vi "shared-dependency-declareself-test.vi"(8 "error in (no error)":errorcluster) -> (0 "error out":errorcluster)   [LabVIEW 2013]
uses:
  _test-support-SMOs/SMO.SelfTerminatingOverride/SMO.SelfTerminatingOverride.lvclass
  src/SMO/SMO.lvclass
  <vilib>/addons/_JKI Toolkits/Caraya/classes/Assert/Assert.lvclass
  <vilib>/addons/_JKI Toolkits/Caraya/classes/Test/Test.lvclass
  src/Registry/Registry-SMO.lvclass
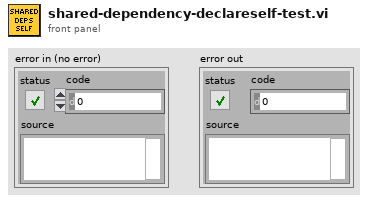
[diagram p1: front panel]
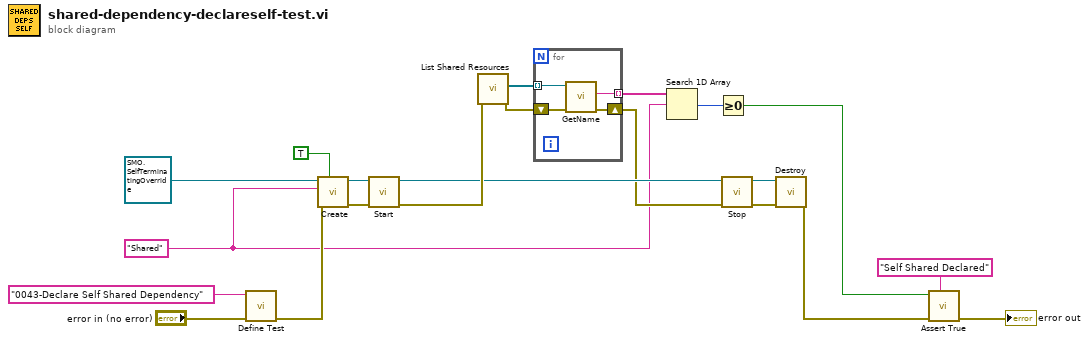
[diagram p0: block diagram]
diagram:
  w4 = "Shared" ("Subsystem Name (optional)")
  n1 = call <vilib>:"Define Test.vi"("error in (no error)"="error in (no error)", "Label (VI Title)"="0043-Declare Self Shared Dependency") -> ("error out"=w13:errorcluster)  [unwired: 9 in]
  n2 = call "Create.vi"("Shared Resource (F)"=TRUE, "error in (no error)"=w13, "Subsystem Name (optional)"=w4, "SMO"=refnum<class "SMO.SelfTerminatingOverride.lvclass"> refnum ("SMO.SelfTerminatingOverride.lvclass")) -> ("error out"=w18:errorcluster, "SMO out"=w17:refnum<class "SMO.SelfTerminatingOverride.lvclass">)  [unwired: 5 in, 1 out]
  n3 = call "Start.vi"("error in (no error)"=w18, "SMO"=w17) -> ("error out"=w9:errorcluster, "SMO out"=w8:refnum<class "SMO.SelfTerminatingOverride.lvclass">)  [unwired: 8 in]
  n4 = call "List Shared Resources.vi"("error in (no error)"=w9) -> ("error out"=w7:errorcluster, "Shared Resources"=w10:refnum<class "SMO.lvclass">[])  [unwired: 9 in]
  n5 = for {
    tunnel: w10 -> [w25] mode=indexing
    tunnel: [w24] -> w5 mode=indexing
    shift-right: [w22] -> w6
    shift-left: w7 -> [w23]
    n6 = call "GetName.vi"("error in (no error)"=w23, "SMO"=w25) -> ("error out"=w22:errorcluster, "Name"=w24:string)  [unwired: 6 in, 2 out]
  }
  n7 = Search 1D Array(1D array=w5, element=w4) -> (index of element=w3:i32)  [unwired: 1 in]
  n8 = Greater Or Equal To 0?(x=w3) -> (x >= 0?=w2:bool)
  n9 = call "Stop.vi"("error in (no error)"=w6, "SMO"=w8) -> ("error out"=w19:errorcluster, "SMO out"=w20:refnum<class "SMO.SelfTerminatingOverride.lvclass">)  [unwired: 8 in]
  n10 = call "Destroy.vi"("error in (no error)"=w19, "SMO"=w20) -> ("error out"=w12:errorcluster)  [unwired: 9 in]
  n11 = call <vilib>:"Assert True.vi"("Label"="Self Shared Declared" ("Filter (regex|name)"), "error in (no error)"=w12, "True?"=w2) -> ("error out"=→"error out":errorcluster)  [unwired: 8 in]
